vi "_ReadTagTemplate.vi"(8 "error in (no error)":errorcluster, 9 "Type":variant, 10 "name":string, 11 "TagMap":refnum<data-value>) -> (0 "error out":errorcluster, 1 "found":bool, 2 "Value":variant, 3 "TagMap(dup)":refnum<data-value>)   [LabVIEW 2017, in "ReadTag.xnode"]
uses:
  ReadTag.xnode
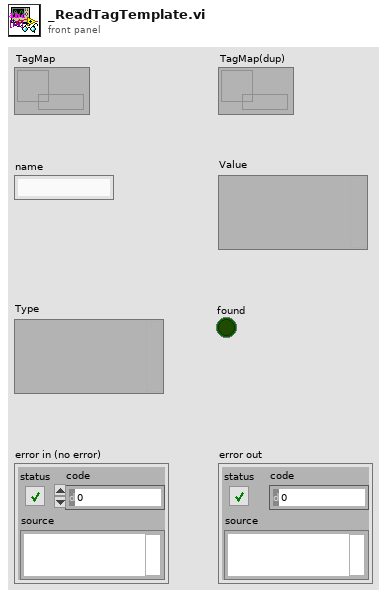
[diagram p1: front panel]
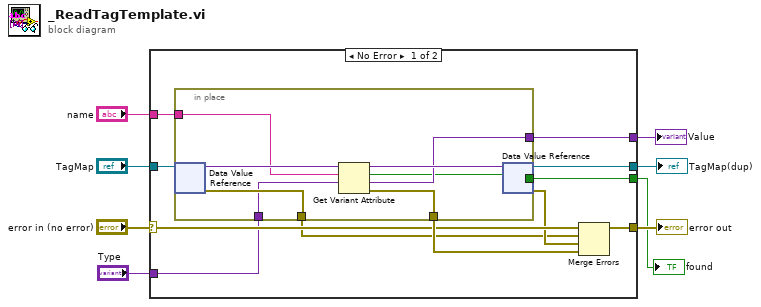
[diagram p0: block diagram]
diagram:
  n1 = case shown="No Error" "error in (no error)" {
    selector: "error in (no error)" -> [w17 w30]
    tunnel: [w18 w30] -> w8
    tunnel: "name" -> [w14 _]
    tunnel: [w13 w29] -> w5
    tunnel: "TagMap" -> [w12 w29]
    tunnel: [w11 w28] -> w3
    tunnel: "Type" -> [w10 w28]
    tunnel: [w9 _] -> w1
    frame No Error {
      n2 = in-place "In Place Element Structure" {
        in-place-border: w14 -> [w25]
        in-place-border: [w23] -> w15
        in-place-border: [w24] -> w19
        in-place-border: [w22] -> w11
        in-place-border: w10 -> [w21]
        in-place-border: [w20] -> w9
        n3 = in-place-dvr #1(w12) -> (w27:variant, w23:errorcluster)
        n4 = Get Variant Attribute(Variant=w27, name=w25, default value (empty Variant)=w21) -> (duplicate Variant=w26:variant, found=w20:bool, value=w22:variant, error out=w24:errorcluster)  [unwired: 1 in]
        n5 = in-place-dvr #1(w26) -> (w13:refnum<data-value>, w16:errorcluster)
      }
      n6 = Merge Errors(w17, w15, w16, w19) -> (w18:errorcluster)
    }
    frame Error {
    }
  }
  "error out" <- w8
  "TagMap(dup)" <- w5
  "Value" <- w3
  "found" <- w1
